vi "Command Timeout.vi"(7 "error source vi name":string, 8 "error in (no error)":errorcluster, 11 "Interface in":refnum<class "Interface.lvclass">) -> (0 "error out":errorcluster, 3 "Interface out":refnum<class "Interface.lvclass">)   [LabVIEW 2019, in "DSF Core.lvlib" / "Interface.lvclass"]
uses:
  Interface.lvclass
  Errors.ctl
  <vilib>/NI/Memory Manager/VIs/New Error Cluster.vi
  <vilib>/NI/Memory Manager/VIs/New Error Cluster (512B).vi
  <vilib>/NI/Memory Manager/VIs/Set Error Code.vi
  <vilib>/NI/Memory Manager/VIs/Set Error Status.vi
  <vilib>/NI/Memory Manager/VIs/Set Error Source.vi
  <vilib>/NI/Memory Manager/VIs/Write String to Source.vi
  Interface Error Info.vi
  VIs/Constants/Constants.vi
  VIs/Constants/Base Error Code.vi
  Interface Error Offset.vi
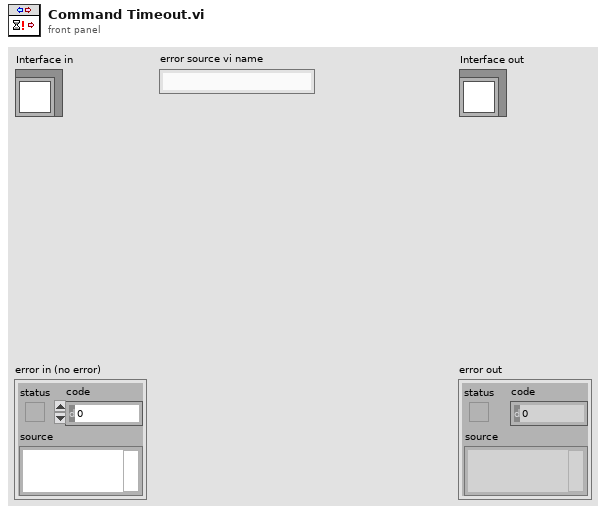
[diagram p1: front panel]
types:
  T1 = typedef "DSF Core.lvlib/Interface.lvclass/Errors.ctl" = enum16{"Command Timeout", "Response Timeout", "Error Timeout", "Invalid Response", "Invalid Response Parameters"}
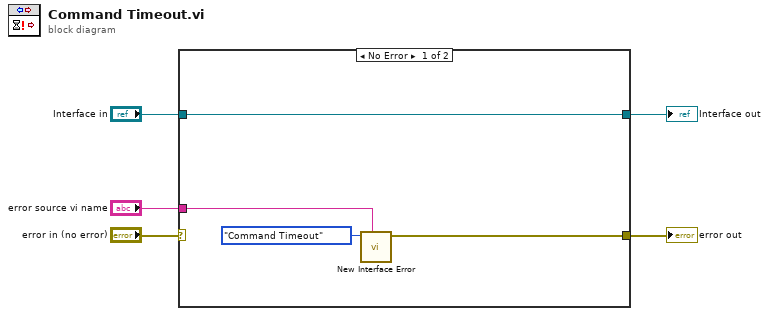
[diagram p0: block diagram]
diagram:
  n1 = case shown="No Error" "error in (no error)" {
    selector: "error in (no error)" -> [_ w10]
    tunnel: "Interface in" -> [w9 w11]
    tunnel: [w9 w11] -> w3
    tunnel: [w8 w10] -> w2
    tunnel: "error source vi name" -> [w7 _]
    frame No Error {
      n2 = call "New Interface Error.vi"("error source vi name"=w7, "error"=Errors."Command Timeout") -> ("error out"=w8:errorcluster)  [unwired: 8 in, 1 out]
    }
    frame Error {
    }
  }
  "error out" <- w2
  "Interface out" <- w3
